vi "Expt8a_MT Convolutional Encode-Decode_Student_lab.vi"() -> ()   [LabVIEW 2020]
doc: "This example demonstrates Convolutional Channel coding and decoding."
uses:
  <vilib>/addons/Modulation/Digital/General/MT Generate Bits (Galois, PN Order).vi
  <vilib>/addons/Modulation/niDMT.lvlib
panel:
  out "Bit Error Rate (no coding)":dbl format="%.4f"
  in  "Initial State":u32 format="%.0x"
  in  "Constraint length":i32=4
  in  "Convolutional Encoder":T1(tab)=enum."Specify Generator Matrix"
  in  "Rate (k/n)":enum16{"1/2", "1/3", "1/4", "2/3", "3/4"}(ring)
  in  "Generator Matrix (n x k)":u32[][](array[numeric])=[[48, 12], [24, 32], [56, 60]] format="%o"
  out "Decoded Bit count":i32
  out "Error Out":errorcluster
  out "Encoded Bit count":i32
  out "Noise":i8[](array[numeric])
  out "Bit Error Rate":dbl
  in  "Noise (bit flip probability)":dbl=0.01 format="%.6g"
  out "Message Bits":i8[](array[numeric])
  out "Encoded Bits":i8[](array[numeric])
  out "Decoded Bits":i8[](array[numeric])
  in  "Message Bits":i32=1000
  # "Convolutional  Code / Decode Programming Example"
  # "Rate 2/3 Generator Matrix"
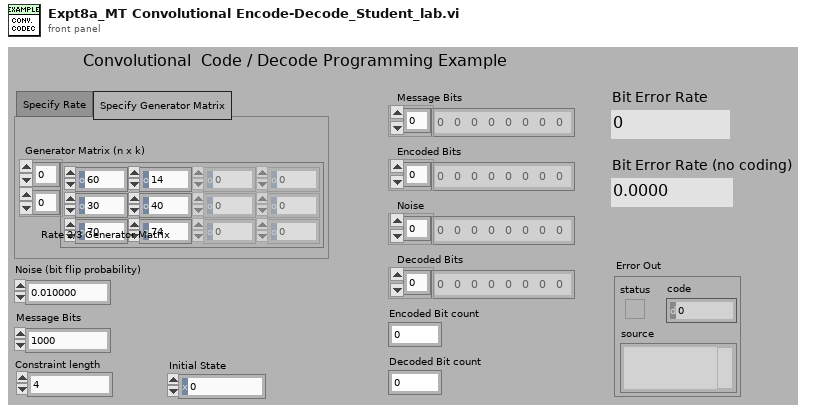
[diagram p1: front panel]
types:
  T1 = enum32{"Specify Rate", "Specify Generator Matrix"}
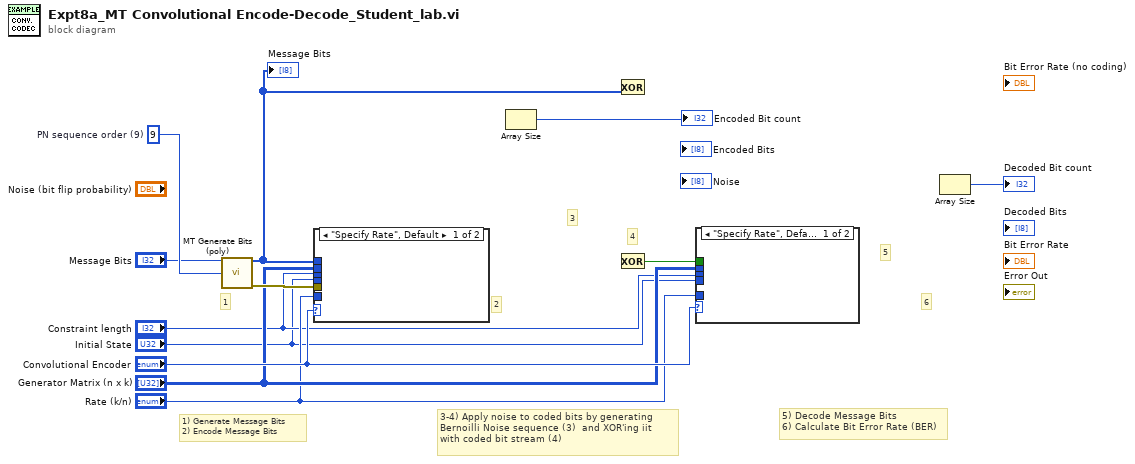
[diagram p0: block diagram]
diagram:
  w11 = 9  # PN sequence order (9)
  # "6"
  # "5"
  # "4"
  # "3"
  # "2"
  # "1"
  # "5) Decode Message Bits\n6) Calculate Bit Error Rate (BER)"
  # "1) Generate Message Bits\n2) Encode Message Bits"
  # "3-4) Apply noise to coded bits by generating \nBernoilli Noise sequence (3)  and XOR'ing iit \nwith coded bit stream (4)"
  n1 = call-poly <vilib>:"MT Generate Bits (poly).vi"("total bits (128)"="Message Bits", "PN sequence order (9)"=w11) -> ("output bit stream"=w1:i8[], "error out"=w9:errorcluster)  [unwired: 11 in, 1 out]
  "Message Bits" <- w1
  n2 = case shown="\"Specify Rate\", Default" "Convolutional Encoder" {
    tunnel: w1 -> [_ _]
    tunnel: w9 -> [_ _]
    tunnel: "Initial State" -> [_ _]
    tunnel: "Constraint length" -> [_ _]
    tunnel: "Rate (k/n)" -> [_ _]
    tunnel: "Generator Matrix (n x k)" -> [_ _]
    frame "Specify Rate", Default {
    }
    frame "Specify Generator Matrix" {
    }
  }
  n3 = Array Size() -> (size(s)=→"Encoded Bit count":i32)  [unwired: 1 in]
  n4 = Exclusive Or(1:w1) -> ()  [unwired: 1 in, 1 out]
  n5 = Exclusive Or() -> (0:w3:bool)  [unwired: 2 in]
  n6 = case shown="\"Specify Rate\", Default" "Convolutional Encoder" {
    tunnel: "Generator Matrix (n x k)" -> [_ _]
    tunnel: "Rate (k/n)" -> [_ _]
    tunnel: "Constraint length" -> [_ _]
    tunnel: "Initial State" -> [_ _]
    tunnel: w3 -> [_ _]
    frame "Specify Rate", Default {
    }
    frame "Specify Generator Matrix" {
    }
  }
  n7 = Array Size() -> (size(s)=→"Decoded Bit count":i32)  [unwired: 1 in]
